vi "Destroy.vi"(8 "error in":errorcluster, 11 "SEQ in":refnum<class "SEQ.lvclass">) -> (0 "error out":errorcluster, 3 "SEQ out":refnum<class "SEQ.lvclass">)   [LabVIEW 2012, in "Sequence Composition.lvlib" / "SEQ.lvclass"]
doc: "Flush the queue containing the steps for the sequence and destroy the reference to the queue."
uses:
  SEQ.lvclass
  SEQ.lvclass/SEQ.ctl
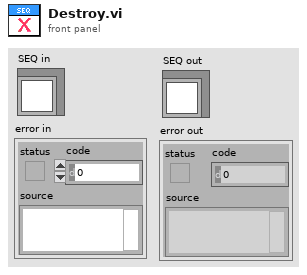
[diagram p1: front panel]
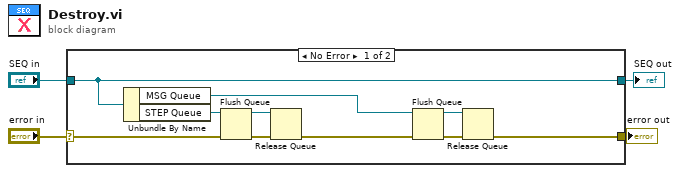
[diagram p0: block diagram]
diagram:
  n1 = case shown="No Error" "error in" {
    selector: "error in" -> [w11 w16]
    tunnel: [w6 w16] -> w3
    tunnel: [w14 w15] -> w1
    tunnel: "SEQ in" -> [w14 w15]
    frame No Error {
      n2 = Unbundle By Name(w14) -> ("MSG Queue"=w5:refnum<queue>, "STEP Queue"=w13:refnum<queue>)
      n3 = Flush Queue(queue=w13, error in (no error)=w11) -> (queue out=w12:refnum<queue>, error out=w10:errorcluster)  [unwired: 1 out]
      n4 = Release Queue(queue=w12, error in (no error)=w10) -> (error out=w7:errorcluster)  [unwired: 1 in, 2 out]
      n5 = Flush Queue(queue=w5, error in (no error)=w7) -> (queue out=w8:refnum<queue>, error out=w9:errorcluster)  [unwired: 1 out]
      n6 = Release Queue(queue=w8, error in (no error)=w9) -> (error out=w6:errorcluster)  [unwired: 1 in, 2 out]
    }
    frame Error {
    }
  }
  "error out" <- w3
  "SEQ out" <- w1
